vi "sub_minmaxmean.vi"(11 "History Data":waveform(dbl)[](array[waveform])) -> (1 "mini":dbl, 2 "max":dbl, 3 "mean":dbl)   [LabVIEW 2013]
uses:
  <vilib>/Analysis/baseanly.llb/Mean (DBL).vi
  <vilib>/Analysis/NI_AALBase.lvlib
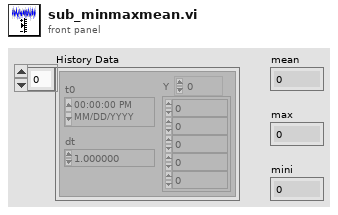
[diagram p1: front panel]
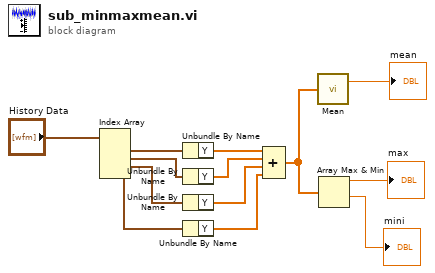
[diagram p0: block diagram]
diagram:
  n1 = Index Array(array="History Data") -> (element #1=w4:waveform(dbl), element #2=w3:waveform(dbl), element #3=w2:waveform(dbl), element #4=w1:waveform(dbl))  [unwired: 4 in]
  n2 = Unbundle By Name(w4) -> ("Y"=w9:dbl[])
  n3 = Unbundle By Name(w3) -> ("Y"=w8:dbl[])
  n4 = Unbundle By Name(w2) -> ("Y"=w7:dbl[])
  n5 = Unbundle By Name(w1) -> ("Y"=w6:dbl[])
  n6 = Compound Arithmetic op=ADD(w9, w8, w7, w6) -> (w10:dbl[])
  n7 = call-poly <vilib>:"Mean.vi"("X"=w10) -> ("mean"=→"mean":dbl)  [unwired: 1 out]
  n8 = Array Max & Min(array=w10) -> (max value=→"max":dbl, min value=→"mini":dbl)  [unwired: 2 out]
